vi "SVN_copy.vi"(8 "error in (no error)":errorcluster, 9 "Message":string, 10 "DestinationURL":string, 11 "SourceURL":string) -> (0 "error out":errorcluster, 1 "command":string, 2 "standard output":string, 3 "standard error":string)   [LabVIEW 2017]
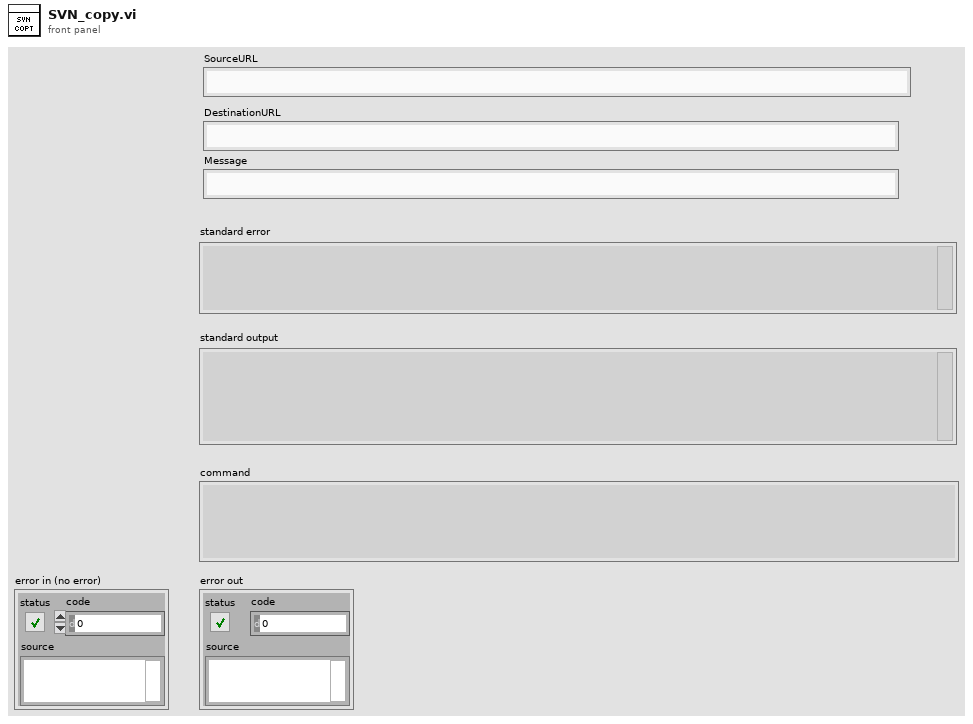
[diagram p1: front panel]
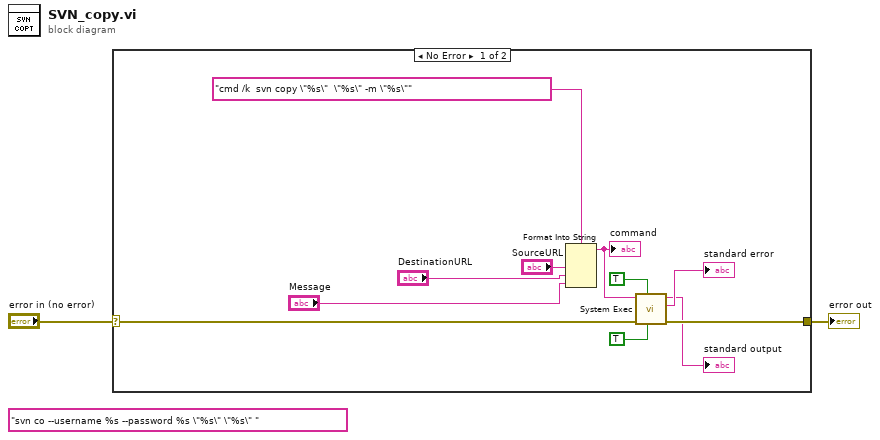
[diagram p0: block diagram]
diagram:
  (unwired) "svn co --username %s --password %s \"%s\" \"%s\" "
  n1 = case shown="No Error" "error in (no error)" {
    selector: "error in (no error)" -> [w12 w14]
    tunnel: [w13 w14] -> w2
    frame No Error {
      n2 = Format Into String(format string="cmd /k  svn copy \"%s\"  \"%s\" -m \"%s\"", "SourceURL", "DestinationURL", "Message") -> (resulting string=w9:string)  [unwired: 2 in, 1 out]
      "command" <- w9
      n3 = call <vilib>:"System Exec.vi"("run minimized? (F)"=TRUE, "wait until completion? (T)"=TRUE, "error in (no error)"=w12, "command line"=w9) -> ("error out"=w13:errorcluster, "standard error"=→"standard error":string, "standard output"=→"standard output":string)  [unwired: 4 in, 1 out]
    }
    frame Error {
    }
  }
  "error out" <- w2
